vi "PPSU Set parameters 2.vi"(8 "Error in":errorcluster, 10 "Data":T1, 11 "Device information":string[](array[string])) -> (0 "Fehler (Ausgang)":errorcluster caption="Error out")   [LabVIEW 2022 SP3]
panel:
  out "Device information out":string[](array[string])
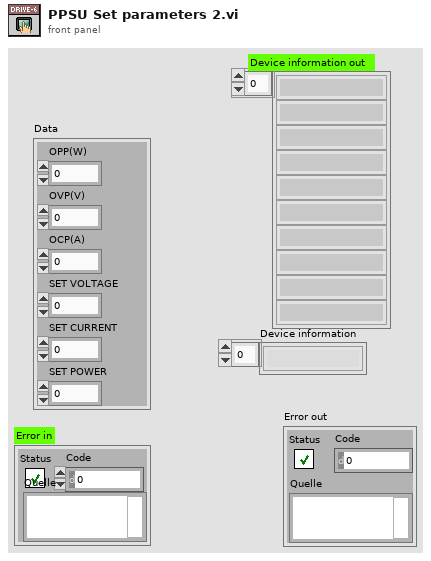
[diagram p1: front panel]
types:
  T1 = cluster{"OPP(W)":dbl, "OVP(V)":dbl, "OCP(A)":dbl, "SET VOLTAGE":dbl, "SET CURRENT":dbl, "SET POWER":dbl}
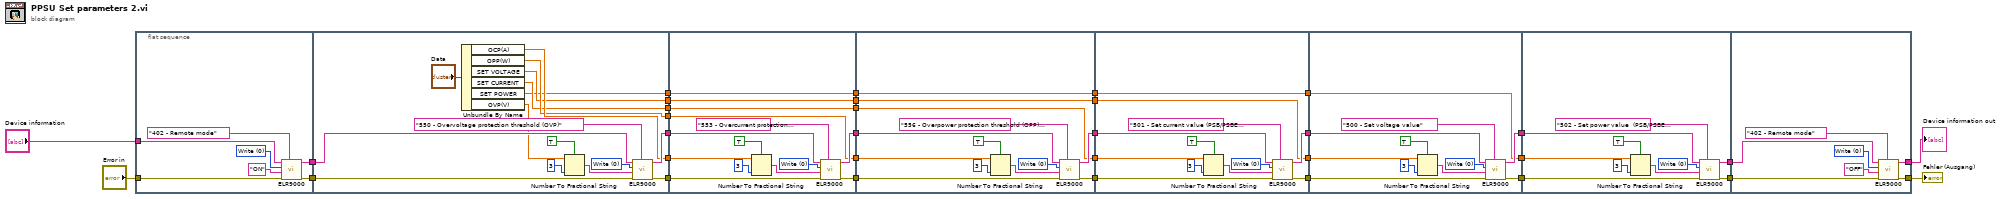
[diagram p0: block diagram]
diagram:
  n1 = flat-sequence {
    tunnel: "Error in" -> [w40]
    tunnel: "Device information" -> [w34]
    tunnel: [w36] -> w33
    tunnel: [w35] -> w32
    tunnel: [w54] -> w31
    tunnel: [w53] -> w30
    tunnel: w33 -> [w52]
    tunnel: w32 -> [w51]
    tunnel: [w47] -> w29
    tunnel: [w46] -> w28
    tunnel: [w45] -> w27
    tunnel: [w44] -> w26
    tunnel: [w43] -> w25
    tunnel: w31 -> [w64]
    tunnel: w30 -> [w65]
    tunnel: [w63] -> w24
    tunnel: [w62] -> w23
    tunnel: w29 -> [w61]
    tunnel: [w60] -> w22
    tunnel: w28 -> [w60]
    tunnel: [w59] -> w21
    tunnel: w27 -> [w59]
    tunnel: [w58] -> w20
    tunnel: w26 -> [w58]
    tunnel: [w57] -> w19
    tunnel: w25 -> [w57]
    tunnel: w24 -> [w78]
    tunnel: w23 -> [w77]
    tunnel: [w76] -> w18
    tunnel: [w75] -> w17
    tunnel: w22 -> [w74]
    tunnel: [w73] -> w16
    tunnel: w21 -> [w73]
    tunnel: [w72] -> w15
    tunnel: w20 -> [w72]
    tunnel: [w71] -> w14
    tunnel: w19 -> [w71]
    tunnel: [w94] -> w13
    tunnel: [w93] -> w12
    tunnel: w18 -> [w88]
    tunnel: w17 -> [w87]
    tunnel: w16 -> [w86]
    tunnel: [w85] -> w11
    tunnel: w15 -> [w85]
    tunnel: [w84] -> w10
    tunnel: w14 -> [w84]
    tunnel: w13 -> [w99]
    tunnel: [w101] -> w9
    tunnel: w12 -> [w98]
    tunnel: [w100] -> w8
    tunnel: w11 -> [w97]
    tunnel: [w96] -> w7
    tunnel: w10 -> [w96]
    tunnel: w9 -> [w111]
    tunnel: [w109] -> w5
    tunnel: w8 -> [w110]
    tunnel: [w108] -> w6
    tunnel: w7 -> [w107]
    tunnel: w6 -> [w123]
    tunnel: w5 -> [w122]
    tunnel: [w118] -> w2
    tunnel: [w117] -> w1
    frame #0 {
      w38 = u8 0 items=["Write", "Read"] ("Access")
      n2 = call <instrlib>:"ELR9000.vi"("Command list"="402 - Remote mode", "Error in"=w40, "Value"="ON", "Access"=w38, "Device information in"=w34) -> ("Error out"=w35:errorcluster, "Device information out"=w36:string[])  [unwired: 1 in, 2 out]
    }
    frame #1 {
      w56 = u8 0 items=["Write", "Read"] ("Access")
      n3 = Unbundle By Name("Data") -> ("OCP(A)"=w47:dbl, "OPP(W)"=w46:dbl, "SET VOLTAGE"=w44:dbl, "SET CURRENT"=w45:dbl, "SET POWER"=w43:dbl, "OVP(V)"=w42:dbl)
      n4 = Number To Fractional String(use system decimal point (T)=TRUE, number=w42, precision (6)=i16 3) -> (F-format string=w48:string)  [unwired: 1 in]
      n5 = call <instrlib>:"ELR9000.vi"("Command list"="550 - Overvoltage protection threshold (OVP)", "Error in"=w51, "Value"=w48, "Access"=w56, "Device information in"=w52) -> ("Error out"=w54:errorcluster, "Device information out"=w53:string[])  [unwired: 1 in, 2 out]
    }
    frame #2 {
      w70 = u8 0 items=["Write", "Read"] ("Access")
      n6 = Number To Fractional String(use system decimal point (T)=TRUE, number=w61, precision (6)=i16 3) -> (F-format string=w66:string)  [unwired: 1 in]
      n7 = call <instrlib>:"ELR9000.vi"("Command list"="553 - Overcurrent protection threshold (OCP) (PSB/PSBE devices: source mode)", "Error in"=w64, "Value"=w66, "Access"=w70, "Device information in"=w65) -> ("Error out"=w62:errorcluster, "Device information out"=w63:string[])  [unwired: 1 in, 2 out]
    }
    frame #3 {
      w83 = u8 0 items=["Write", "Read"] ("Access")
      n8 = Number To Fractional String(use system decimal point (T)=TRUE, number=w74, precision (6)=i16 3) -> (F-format string=w79:string)  [unwired: 1 in]
      n9 = call <instrlib>:"ELR9000.vi"("Command list"="556 - Overpower protection threshold (OPP) (PSB/PSBE devices: source mode)", "Error in"=w77, "Value"=w79, "Access"=w83, "Device information in"=w78) -> ("Error out"=w75:errorcluster, "Device information out"=w76:string[])  [unwired: 1 in, 2 out]
    }
    frame #4 {
      w95 = u8 0 items=["Write", "Read"] ("Access")
      n10 = Number To Fractional String(use system decimal point (T)=TRUE, number=w86, precision (6)=i16 3) -> (F-format string=w89:string)  [unwired: 1 in]
      n11 = call <instrlib>:"ELR9000.vi"("Command list"="501 - Set current value (PSB/PSBE devices: source mode) / Irradiation (PV function, PSI/PSB only) ", "Error in"=w87, "Value"=w89, "Access"=w95, "Device information in"=w88) -> ("Error out"=w93:errorcluster, "Device information out"=w94:string[])  [unwired: 1 in, 2 out]
    }
    frame #5 {
      w106 = u8 0 items=["Write", "Read"] ("Access")
      n12 = Number To Fractional String(use system decimal point (T)=TRUE, number=w97, precision (6)=i16 3) -> (F-format string=w102:string)  [unwired: 1 in]
      n13 = call <instrlib>:"ELR9000.vi"("Command list"="500 - Set voltage value", "Error in"=w98, "Value"=w102, "Access"=w106, "Device information in"=w99) -> ("Error out"=w100:errorcluster, "Device information out"=w101:string[])  [unwired: 1 in, 2 out]
    }
    frame #6 {
      w116 = u8 0 items=["Write", "Read"] ("Access")
      n14 = Number To Fractional String(use system decimal point (T)=TRUE, number=w107, precision (6)=i16 3) -> (F-format string=w112:string)  [unwired: 1 in]
      n15 = call <instrlib>:"ELR9000.vi"("Command list"="502 - Set power value  (PSB/PSBE devices: source mode)", "Error in"=w110, "Value"=w112, "Access"=w116, "Device information in"=w111) -> ("Error out"=w108:errorcluster, "Device information out"=w109:string[])  [unwired: 1 in, 2 out]
    }
    frame #7 {
      w120 = u8 0 items=["Write", "Read"] ("Access")
      n16 = call <instrlib>:"ELR9000.vi"("Command list"="402 - Remote mode", "Error in"=w123, "Value"="OFF", "Access"=w120, "Device information in"=w122) -> ("Error out"=w117:errorcluster, "Device information out"=w118:string[])  [unwired: 1 in, 2 out]
    }
  }
  "Device information out" <- w2
  "Fehler (Ausgang)" <- w1
